vi "Read.vi"(8 "error in (no error)":errorcluster caption="错误输入（无错误）", 11 "2700 输入":refnum<class "2700.lvclass">) -> (0 "error out":errorcluster caption="错误输出", 2 "Measurement Data":dbl[](array[numeric]), 3 "2700 输出":refnum<class "2700.lvclass">)   [LabVIEW 2021, in "2700.lvclass"]
uses:
  2700.lvclass
  2700.lvclass/2700.ctl
  <instrlib>/Keithley 27XX/Public/Data/Read Multiple Direct.vi
  <instrlib>/Keithley 27XX/Keithley 27XX.lvlib
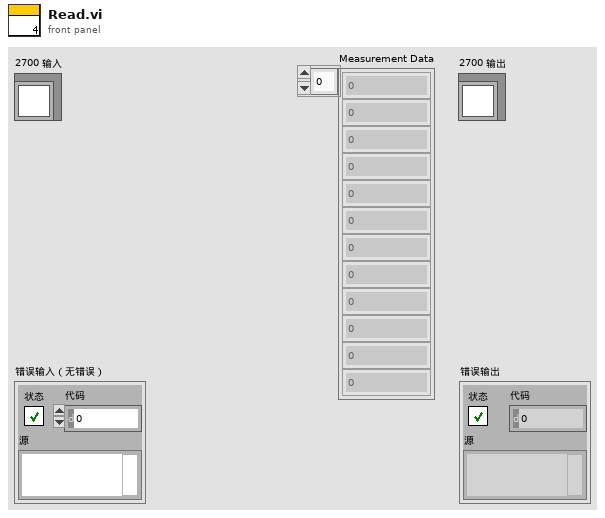
[diagram p1: front panel]
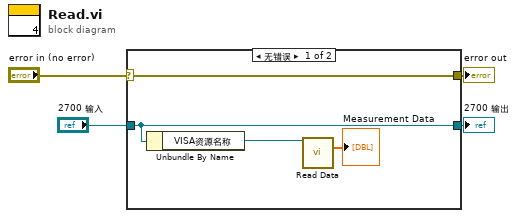
[diagram p0: block diagram]
diagram:
  n1 = case shown="无错误" "error in (no error)" {
    selector: "error in (no error)" -> [w7 w9]
    tunnel: "2700 输入" -> [w6 w10]
    tunnel: [w7 w9] -> w2
    tunnel: [w6 w10] -> w1
    frame No Error {
      n2 = Unbundle By Name(w6) -> ("VISA资源名称"=w8:refnum<visa-resource-name>)
      n3 = call-poly <instrlib>:"Read Data.vi"("VISA resource name"=w8) -> ("Measurement Data"=→"Measurement Data":dbl[])  [unwired: 9 in, 5 out]
    }
    frame Error {
    }
  }
  "error out" <- w2
  "2700 输出" <- w1
